vi "Data Point Filter.vi"(10 "Data Points":T2(array[cluster])) -> (2 "Filtered Data":T1(array[cluster]))   [LabVIEW 2017]
panel:
  out "New Data Points":T1(array[cluster])
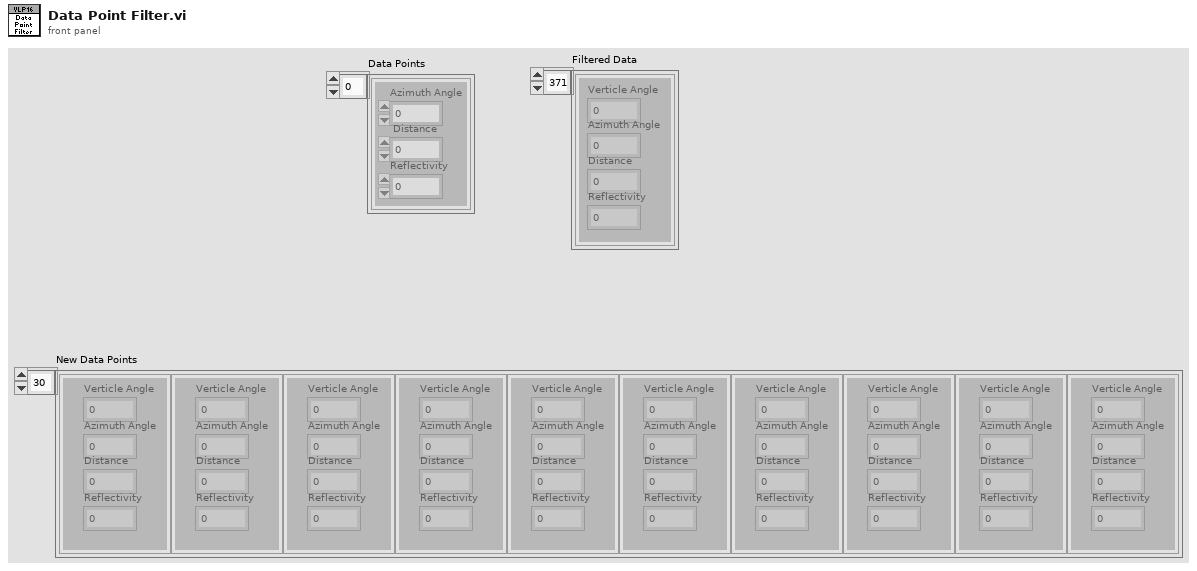
[diagram p1: front panel]
types:
  T1 = cluster{"Verticle Angle":dbl, "Azimuth Angle":dbl, "Distance":dbl, "Reflectivity":dbl}[]
  T2 = cluster{"Azimuth Angle":dbl, " Distance":dbl, "Reflectivity":dbl}[]
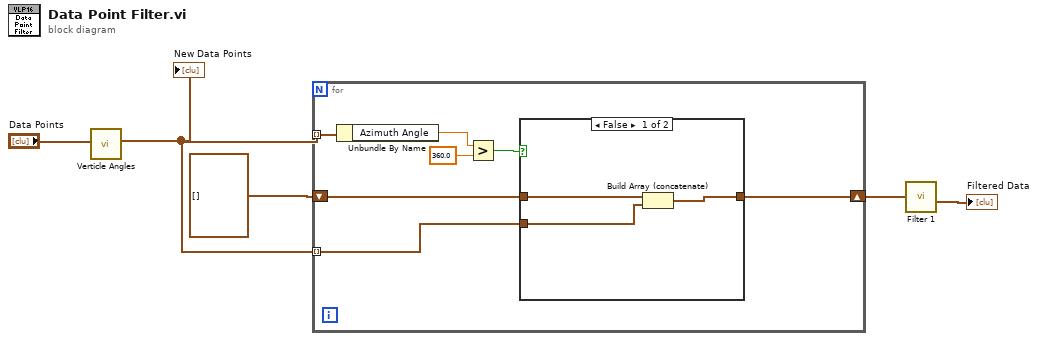
[diagram p0: block diagram]
diagram:
  n1 = call "Verticle Angles.vi"("Data Points"="Data Points") -> ("New Data Points"=w5:T1)  [unwired: 10 in]
  "New Data Points" <- w5
  n2 = for {
    tunnel: w5 -> [w12] mode=indexing
    shift-right: [w7] -> w4
    shift-left: cluster{dbl, dbl, dbl, dbl}[] [] -> [w8]
    tunnel: w5 -> [w6] mode=indexing
    n3 = Unbundle By Name(w12) -> ("Azimuth Angle"=w11:dbl)
    n4 = Greater?(x=w11, y=360.0) -> (0:w9:bool)
    n5 = case shown="False" w9 {
      tunnel: w8 -> [w15 w16]
      tunnel: [w14 w16] -> w7
      tunnel: w6 -> [w13 _]
      frame False {
        n6 = Build Array (concatenate)(w15, w13) -> (w14:T1)
      }
      frame True {
      }
    }
  }
  n7 = call "Filter 1.vi"("Data for Filtering"=w4) -> ("Filtered Data"=→"Filtered Data":T1)  [unwired: 10 in]
